vi "Config GSM Pattern.vi"(0 "VISA Resource Name":refnum<visa-resource-name>, 1 "Pattern Trigger (2:TRIG KEY)":enum16{"BUS", "EXTERNAL", "TRIGGER KEY"}(ring)=enum."TRIGGER KEY", 2 "Ext Delay (F:OFF)":bool, 3 "Ext Delay Bits (0)":i32, 5 "Pattern Repeat (F:CONT)":bool, 7 "Data (0:PN9)":T1(ring), 9 "FIX4 (0000)":i16 format="%.0b", 11 "error in (no error)":errorcluster {"code" format="%.0x"}, 12 "User File Name (BIN_DATA)":string="BIN_DATA") -> (4 "VISA Resource Name Out":refnum<visa-resource-name>, 15 "error out":errorcluster {"code" format="%.0x"})   [LabVIEW 2012, in "Agilent ESG Series.lvlib"]
doc: "This VI is used to configure GSM pattern data."
uses:
  <instrlib>/Agilent ESG Series/Agilent ESG Series.lvlib
panel:
  # "SINGLE"
  # "CONT"
  # "ON"
  # "OFF"
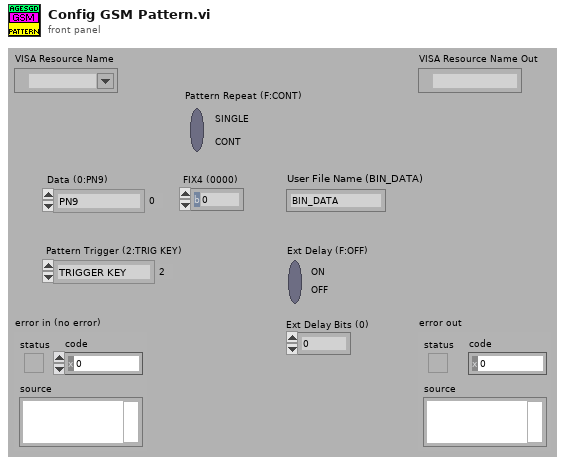
[diagram p1: front panel]
types:
  T1 = enum16{"PN9", "PN15", "FIX4", "USER FILE", "EXT", "4 1's & 4 0's", "8 1's & 8 0's", "16 1's & 16 0's", "32 1's & 32 0's", "64 1's & 64 0's"}
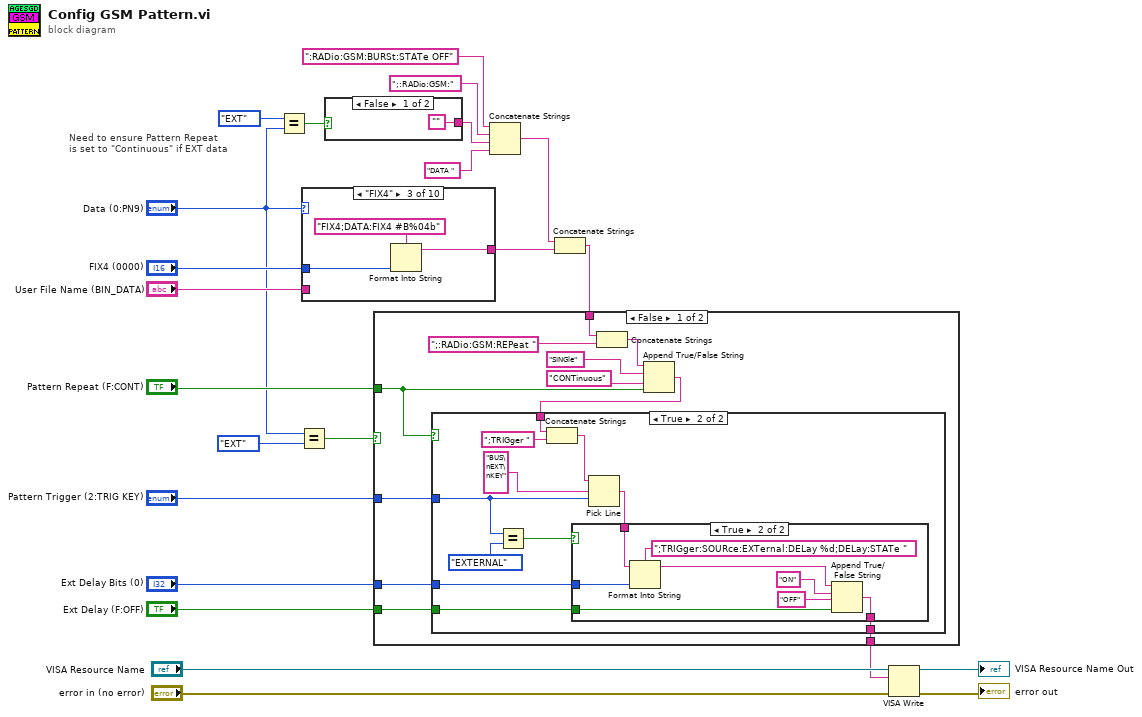
[diagram p0: block diagram]
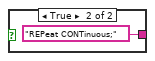
[diagram p2: hidden frame]
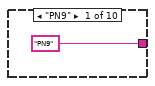
[diagram p3: hidden frame]
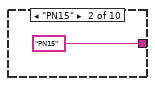
[diagram p4: hidden frame]
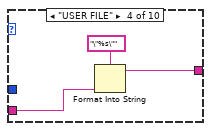
[diagram p5: hidden frame]
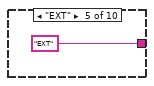
[diagram p6: hidden frame]
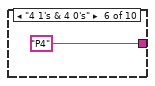
[diagram p7: hidden frame]
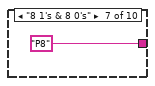
[diagram p8: hidden frame]
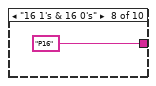
[diagram p9: hidden frame]
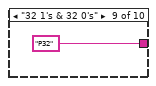
[diagram p10: hidden frame]
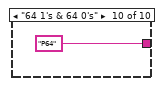
[diagram p11: hidden frame]
diagram:
  # "Need to ensure Pattern Repeat \nis set to \"Continuous\" if EXT data"
  n1 = Equal?(x=T1."EXT" ("y"), y="Data (0:PN9)") -> (x = y?=w5:bool)
  n2 = Equal?(x="Data (0:PN9)", y=T1."EXT") -> (x = y?=w13:bool)
  n3 = case shown="\"FIX4\"" "Data (0:PN9)" {
    tunnel: ["PN9" "PN15" w27 w30 "EXT" "P4" "P8" "P16" "P32" "P64"] -> w18
    tunnel: "FIX4 (0000)" -> [_ _ w26 _ _ _ _ _ _ _]
    tunnel: "User File Name (BIN_DATA)" -> [_ _ _ w29 _ _ _ _ _ _]
    frame "PN9" {
    }
    frame "PN15" {
    }
    frame "FIX4" {
      n4 = Format Into String(format string="FIX4;DATA:FIX4 #B%04b", w26) -> (resulting string=w27:string)  [unwired: 2 in, 1 out]
    }
    frame "USER FILE" {
      n5 = Format Into String(format string="\"%s\"", w29) -> (resulting string=w30:string)  [unwired: 2 in, 1 out]
    }
    frame "EXT" {
    }
    frame "4 1's & 4 0's" {
    }
    frame "8 1's & 8 0's" {
    }
    frame "16 1's & 16 0's" {
    }
    frame "32 1's & 32 0's" {
    }
    frame "64 1's & 64 0's" {
    }
  }
  n6 = case shown="False" w5 {
    tunnel: ["" "REPeat CONTinuous;"] -> w6
    frame False {
    }
    frame True {
    }
  }
  n7 = Concatenate Strings(":RADio:GSM:BURSt:STATe OFF", ";:RADio:GSM:", w6, "DATA ") -> (w7:string)
  n8 = Concatenate Strings(w7, w18) -> (w15:string)
  n9 = case shown="False" w13 {
    tunnel: w15 -> [w44 w72]
    tunnel: "Pattern Trigger (2:TRIG KEY)" -> [w45 _]
    tunnel: "Ext Delay (F:OFF)" -> [w48 _]
    tunnel: [w47 w72] -> w8
    tunnel: "Ext Delay Bits (0)" -> [w46 _]
    tunnel: "Pattern Repeat (F:CONT)" -> [w40 _]
    frame False {
      n10 = Concatenate Strings(w44, ";:RADio:GSM:REPeat ") -> (w49:string)
      n11 = Append True/False String(1:w40, 2:"CONTinuous" ("false string"), 3:"SINGle" ("true string"), 4:w49) -> (0:w43:string)
      n12 = case shown="True" w40 {
        tunnel: w43 -> [w51 w60]
        tunnel: w45 -> [_ w54]
        tunnel: w46 -> [_ w59]
        tunnel: [w51 w58] -> w47
        tunnel: w48 -> [_ w57]
        frame False {
        }
        frame True {
          n13 = Equal?(x=w54, y=enum16{"BUS", "EXTERNAL", "TRIGGER KEY"}."EXTERNAL") -> (x = y?=w52:bool)
          n14 = Concatenate Strings(w60, ";TRIGger ") -> (w62:string)
          n15 = Pick Line(string ("")=w62, multi-line string="BUS\nEXT\nKEY", line index=w54) -> (output string=w56:string)
          n16 = case shown="True" w52 {
            tunnel: w56 -> [w63 w71]
            tunnel: w57 -> [_ w70]
            tunnel: [w63 w69] -> w58
            tunnel: w59 -> [_ w68]
            frame False {
            }
            frame True {
              n17 = Format Into String(format string=";TRIGger:SOURce:EXTernal:DELay %d;DELay:STATe ", initial string=w71, w68) -> (resulting string=w67:string)  [unwired: 1 in, 1 out]
              n18 = Append True/False String(1:w70, 2:"OFF" ("false string"), 3:"ON" ("true string"), 4:w67) -> (0:w69:string)
            }
          }
        }
      }
    }
    frame True {
    }
  }
  n19 = VISA Write(VISA resource name="VISA Resource Name", write buffer=w8, error in (no error)="error in (no error)") -> (VISA resource name out=→"VISA Resource Name Out":refnum<visa-resource-name>, error out=→"error out":errorcluster)  [unwired: 1 out]
